vi "Numbers2Strings.vi"(4 "Number 4":dbl format="%#_13g", 5 "Number 3":dbl format="%#_13g", 6 "Number 2":dbl format="%#_13g", 7 "Number":dbl format="%#_13g") -> (0 "Numeric String 4":string, 1 "Numeric String 3":string, 2 "Numeric String 2":string, 3 "Numeric String 1":string)   [LabVIEW 2018]
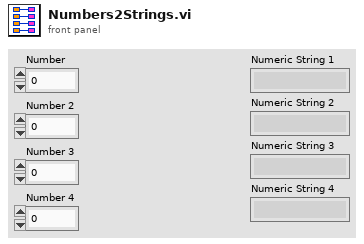
[diagram p1: front panel]
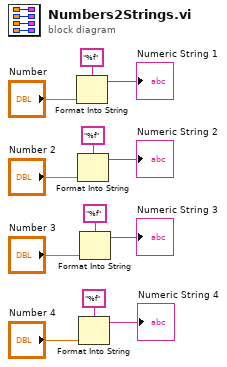
[diagram p0: block diagram]
diagram:
  n1 = Format Into String(format string="%f", "Number") -> (resulting string=→"Numeric String 1":string)  [unwired: 2 in, 1 out]
  n2 = Format Into String(format string="%f", "Number 2") -> (resulting string=→"Numeric String 2":string)  [unwired: 2 in, 1 out]
  n3 = Format Into String(format string="%f", "Number 4") -> (resulting string=→"Numeric String 4":string)  [unwired: 2 in, 1 out]
  n4 = Format Into String(format string="%f", "Number 3") -> (resulting string=→"Numeric String 3":string)  [unwired: 2 in, 1 out]
